vi "Day 11 Puzzle 1.vi"(11 "Path":path) -> ()   [LabVIEW 2021]
uses:
  2502efef-52cf-4e36-8a2b-24fad6cf7fcc.vi
  <vilib>/Utility/file.llb/Read Delimited Spreadsheet (string).vi
  <vilib>/Comparison/Less/Less Functor/Less Functor.lvclass
panel:
  out "Monkey business":i32
  out "Array 3":i32[](array[numeric])
  out "length":i32
  out "deleted portion":string[](array[string])
  out "array w/ subset deleted":string[](array[string])
  out "all rows":string[][](array[string])
  out "subarray":string[](array[string])
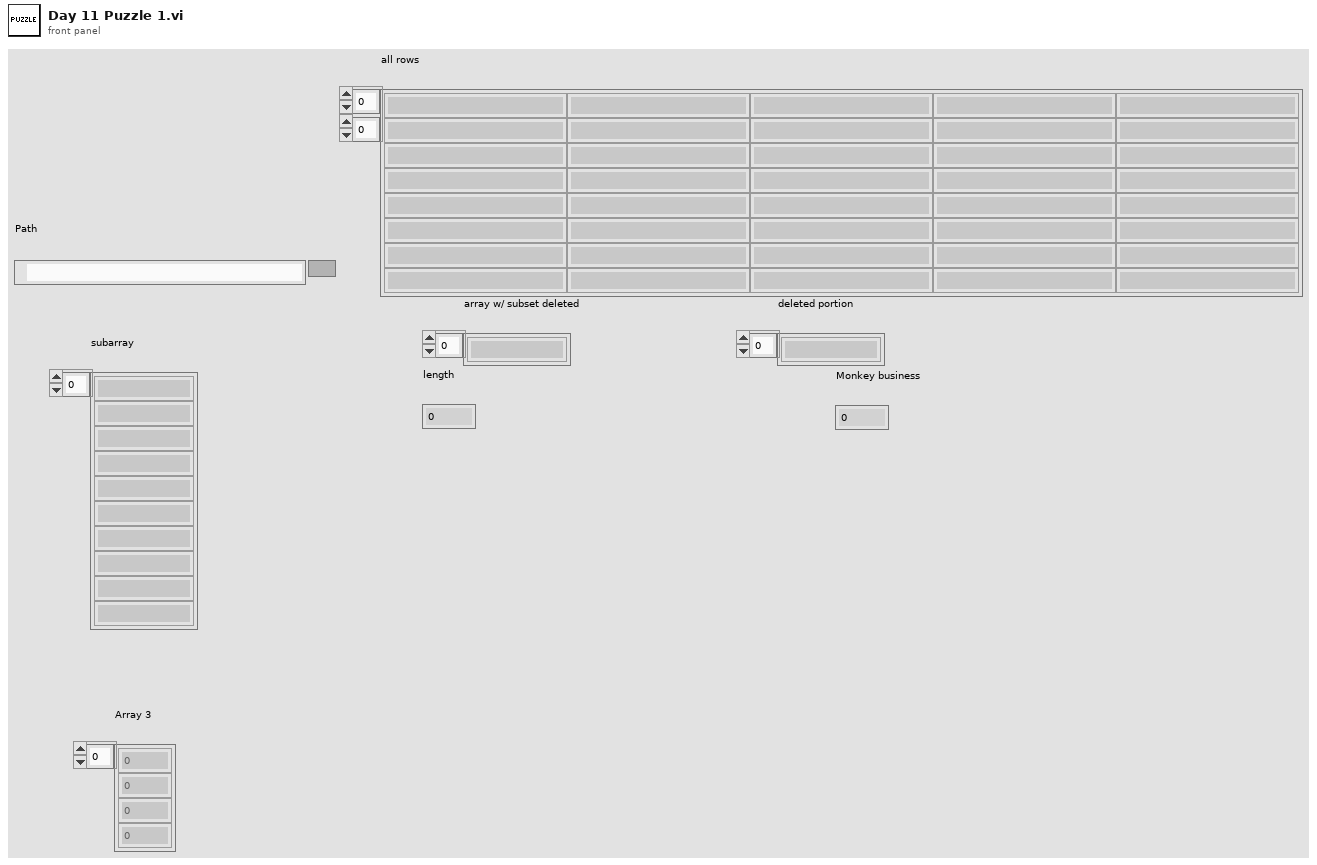
[diagram p1: front panel]
types:
  T1 = cluster{"Items":i32[], "Operation":string, "Operation argument":string, "Divisible by?":i32, "If true":i32, "If false":i32, "Number of inspections":i32}
  T2 = cluster{"Items":i32[], "Operation":string, "Operation argument":string, "Divisible by?":i32, "If true":i32, "If false":i32, "Number of inspections":i32}[]
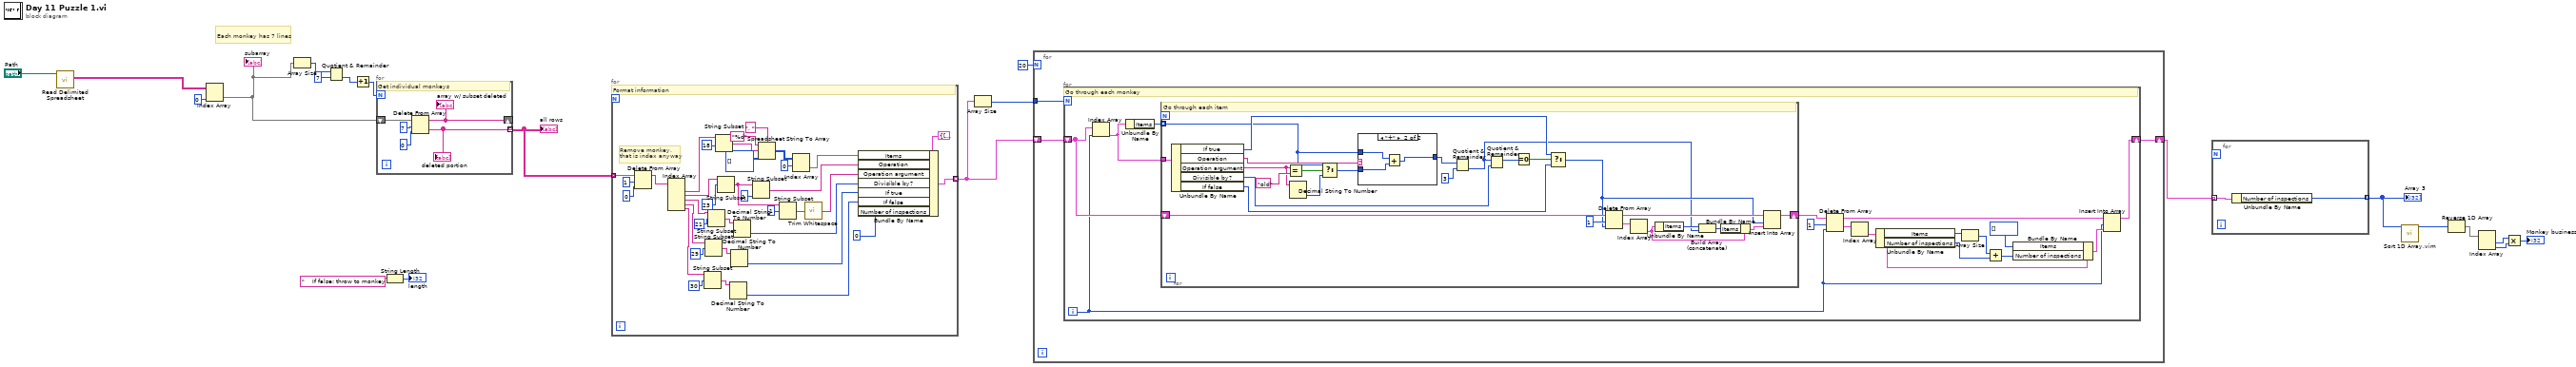
[diagram p0: block diagram]
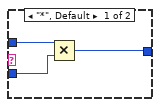
[diagram p2: hidden frame]
diagram:
  # "Each monkey has 7 lines"
  n1 = call-poly <vilib>:"Read Delimited Spreadsheet.vi"("file path (dialog if empty)"="Path") -> ("all rows"=w21:string[][])  [unwired: 9 in, 5 out]
  n2 = Index Array(array=w21, index (col)=0 ("disabled index (col)")) -> (element=w18:string[])  [unwired: 1 in]
  "subarray" <- w18
  n3 = Array Size(array=w18) -> (size(s)=w17:i32)
  n4 = Quotient & Remainder(x=w17, y=7) -> (floor(x/y)=w15:i32)  [unwired: 1 out]
  n5 = Increment(x=w15) -> (x+1=w14:i32)
  n6 = for {
    N: w14 -> [_]
    shift-right: [w23] -> _
    shift-left: w18 -> [w26]
    tunnel: [w22] -> w13 mode=indexing
    # "Get individual monkeys"
    n7 = Delete From Array(array=w26, length=7 ("index"), index=0 ("length")) -> (deleted portion=w22:string[], array with subset deleted=w23:string[])
    "array w/ subset deleted" <- w23
    "deleted portion" <- w22
  }
  "all rows" <- w13
  n8 = String Length(string="    If false: throw to monkey ") -> (length=→"length":i32)
  n9 = for {
    tunnel: w13 -> [w62] mode=indexing
    tunnel: [w28] -> w9 mode=indexing
    # "Remove monkey, \nthat is index anyway"
    # "Format information"
    n10 = Delete From Array(array=w62, length=1, index=0) -> (array with subset deleted=w59:string[])  [unwired: 1 out]
    n11 = Index Array(array=w59) -> (element #1=w58:string, element #2=w49:string, element #3=w40:string, element #4=w35:string, element #5=w32:string)  [unwired: 5 in]
    n12 = String Subset(string=w32, offset (0)=30) -> (substring=w33:string)  [unwired: 1 in]
    n13 = String Subset(string=w35, offset (0)=29) -> (substring=w36:string)  [unwired: 1 in]
    n14 = String Subset(string=w40, offset (0)=21) -> (substring=w39:string)  [unwired: 1 in]
    n15 = String Subset(string=w58, offset (0)=18) -> (substring=w54:string)  [unwired: 1 in]
    n16 = String Subset(string=w49, offset (0)=23) -> (substring=w45:string)  [unwired: 1 in]
    n17 = Decimal String To Number(string=w33) -> (number=w30:i32)  [unwired: 2 in, 1 out]
    n18 = Decimal String To Number(string=w36) -> (number=w31:i32)  [unwired: 2 in, 1 out]
    n19 = Decimal String To Number(string=w39) -> (number=w38:i32)  [unwired: 2 in, 1 out]
    n20 = String Subset(string=w45, length (rest)=1 ("length (rest)")) -> (substring=w46:string)  [unwired: 1 in]
    n21 = Spreadsheet String To Array(delimiter (Tab)=", ", format string="%d", spreadsheet string=w54, array type (2D Dbl)=i32[][] []) -> (array=w52:i32[][])
    n22 = String Subset(string=w45, offset (0)=1) -> (substring=w43:string)  [unwired: 1 in]
    n23 = Index Array(array=w52, index (row)=0) -> (element=w50:i32[])  [unwired: 1 in]
    n24 = call <vilib>:"Trim Whitespace.vi"("string"=w43) -> ("trimmed string"=w42:string)  [unwired: 1 in]
    n25 = Bundle By Name(cluster=T1 {"Items"=[], "Operation"="", "Operation argument"="", "Divisible by?"=0, "If true"=0, "If false"=0, "Number of inspections"=0} ("output cluster"), "Items"=w50, "Operation"=w46, "Operation argument"=w42, "Divisible by?"=w38, "If true"=w31, "If false"=w30, "Number of inspections"=0) -> (w28:T1)
  }
  n26 = Array Size(array=w9) -> (size(s)=w10:i32)
  n27 = for {
    N: 20 -> [_]
    tunnel: w10 -> [w65]
    shift-right: [w63] -> w7
    shift-left: w9 -> [w64]
    n28 = for {
      N: w65 -> [_]
      shift-right: [w71] -> w63
      shift-left: w64 -> [w79]
      i -> [w72]
      # "Go through each monkey"
      n29 = Index Array(array=w79, index=w72) -> (element=w80:T1)
      n30 = Unbundle By Name(w80) -> ("Items"=w81:i32[])
      n31 = for {
        tunnel: w81 -> [w91] mode=indexing
        tunnel: w80 -> [w107]
        shift-right: [w85] -> w74
        shift-left: w79 -> [w95]
        # "Go through each item"
        n32 = Unbundle By Name(w107) -> ("If true"=w97:i32, "Operation"=w106:string, "Operation argument"=w103:string, "Divisible by?"=w100:i32, "If false"=w96:i32)
        n33 = Equal?(x=w103, y="old") -> (x = y?=w104:bool)
        n34 = Decimal String To Number(string=w103) -> (number=w102:i32)  [unwired: 2 in, 1 out]
        n35 = Select(t=w91, s=w104, f=w102) -> (s? t:f=w101:i32)
        n36 = case shown="\"+\"" w106 {
          tunnel: w101 -> [w109 w113]
          tunnel: w91 -> [w110 w112]
          tunnel: [w108 w111] -> w84
          frame "*", Default {
            n37 = Multiply(x=w110, y=w109) -> (x*y=w108:i32)
          }
          frame "+" {
            n38 = Add(x=w112, y=w113) -> (x+y=w111:i32)
          }
        }
        n39 = Quotient & Remainder(x=w84, y=3) -> (floor(x/y)=w82:i32)  [unwired: 1 out]
        n40 = Quotient & Remainder(x=w82, y=w100) -> (x-y*floor(x/y)=w99:i32)  [unwired: 1 out]
        n41 = Equal To 0?(x=w99) -> (x = 0?=w98:bool)
        n42 = Select(t=w97, s=w98, f=w96) -> (s? t:f=w87:i32)
        n43 = Delete From Array(array=w95, length=1, index=w87) -> (deleted portion=w93:T2, array with subset deleted=w88:T2)
        n44 = Index Array(array=w93) -> (element=w90:T1)  [unwired: 1 in]
        n45 = Unbundle By Name(w90) -> ("Items"=w92:i32[])
        n46 = Build Array (concatenate)(w92, w82) -> (w89:i32[])
        n47 = Bundle By Name(cluster=w90, "Items"=w89) -> (w86:T1)
        n48 = Insert Into Array(array=w88, index=w87, new element=w86) -> (w85:T2)
      }
      n49 = Delete From Array(array=w74, length=1, index=w72) -> (deleted portion=w77:T2, array with subset deleted=w76:T2)
      n50 = Index Array(array=w77) -> (element=w70:T1)  [unwired: 1 in]
      n51 = Unbundle By Name(w70) -> ("Items"=w69:i32[], "Number of inspections"=w67:i32)
      n52 = Array Size(array=w69) -> (size(s)=w68:i32)
      n53 = Add(x=w68, y=w67) -> (x+y=w66:i32)
      n54 = Bundle By Name(cluster=w70, "Items"=i32[] [], "Number of inspections"=w66) -> (w75:T1)
      n55 = Insert Into Array(array=w76, index=w72, new element=w75) -> (w71:T2)
    }
  }
  n56 = for {
    tunnel: w7 -> [w115] mode=indexing
    tunnel: [w114] -> w6 mode=indexing
    n57 = Unbundle By Name(w115) -> ("Number of inspections"=w114:i32)
  }
  "Array 3" <- w6
  n58 = call "Sort 1D Array.vim"("unsorted array"=w6) -> ("sorted array"=w5:i32[])  [unwired: 10 in]
  n59 = Reverse 1D Array(array=w5) -> (reversed array=w4:i32[])
  n60 = Index Array(array=w4) -> (element #1=w3:i32, element #2=w2:i32)  [unwired: 2 in]
  n61 = Multiply(x=w3, y=w2) -> (x*y=→"Monkey business":i32)
